vi "SetOutputState.vi"(8 "Error In":errorcluster, 9 "Enabled?":bool, 10 "Output Channel (1 or 2)":u8=1 min=1 max=2 step=1, 11 "Keithley 6482 In":refnum<visa-resource-name>) -> (0 "Error Out":errorcluster, 3 "Keithley 6482 Out":refnum<visa-resource-name>)   [LabVIEW 2010, in "Keithley-6482-Visa.lvlib"]
uses:
  <instrlib>/lib-labview-8.6-export/Keithley-6482-Visa.lvlib
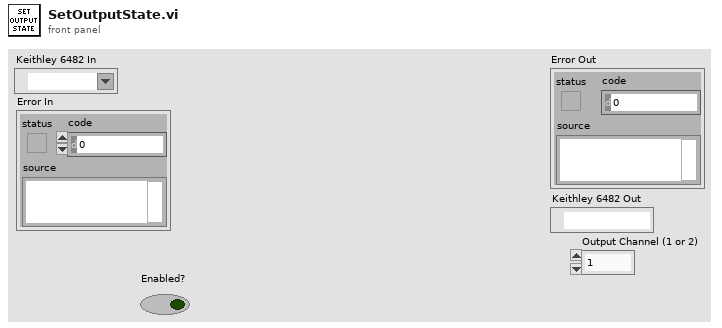
[diagram p1: front panel]
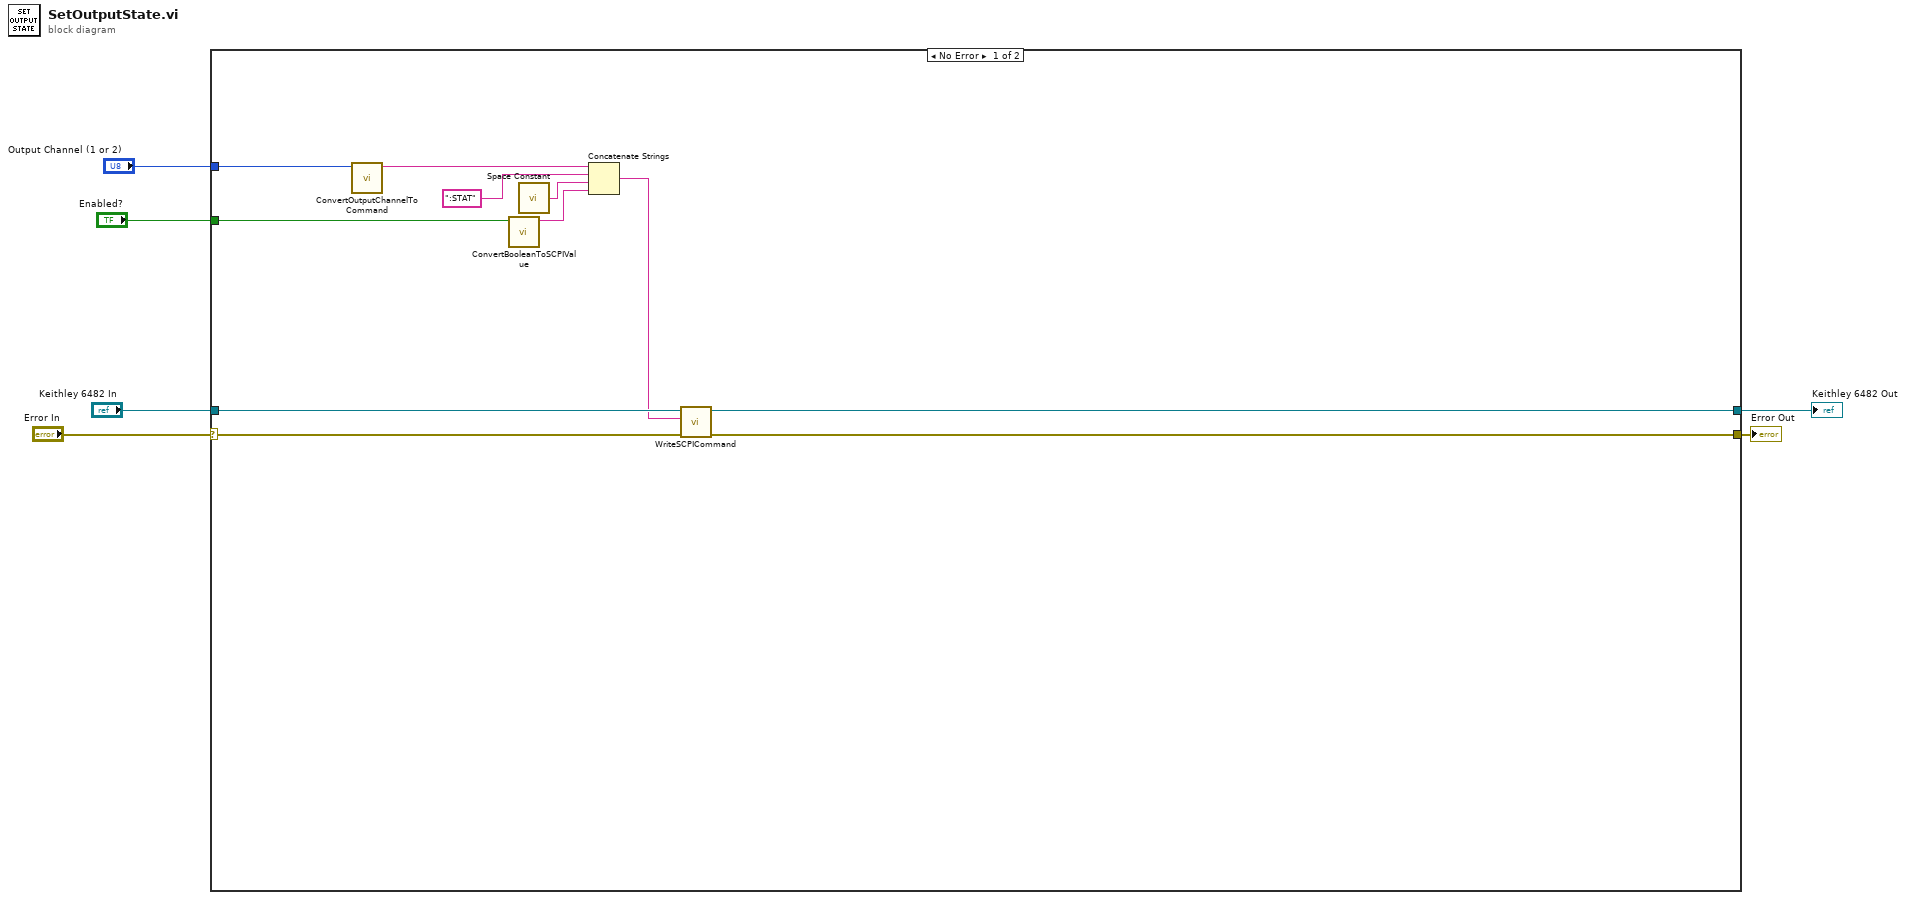
[diagram p0: block diagram]
diagram:
  n1 = case shown="No Error" "Error In" {
    selector: "Error In" -> [w11 w18]
    tunnel: "Keithley 6482 In" -> [w14 w19]
    tunnel: [w12 w18] -> w4
    tunnel: [w13 w19] -> w3
    tunnel: "Enabled?" -> [w17 _]
    tunnel: "Output Channel (1 or 2)" -> [w7 _]
    frame No Error {
      n2 = call <instrlib>:"ConvertOutputChannelToCommand.vi"("Output Channel (1 or 2)"=w7) -> ("Command"=w9:string)  [unwired: 10 in]
      n3 = call <instrlib>:"ConvertBooleanToSCPIValue.vi"("Boolean"=w17) -> ("SCPI Value"=w15:string)  [unwired: 10 in]
      n4 = call <vilib>:"Space Constant.vi"() -> ("String"=w16:string)
      n5 = Concatenate Strings(w9, ":STAT" ("string"), w16, w15) -> (w10:string)
      n6 = call <instrlib>:"WriteSCPICommand.vi"("Error In"=w11, "SCPI Command"=w10, "Keithley 6482 In"=w14) -> ("Error Out"=w12:errorcluster, "Keithley 6482 Out"=w13:refnum<visa-resource-name>)  [unwired: 7 in]
    }
    frame Error {
    }
  }
  "Error Out" <- w4
  "Keithley 6482 Out" <- w3
